vi "lvEtherbone.device_write_single.vi"(0 "eb_socketID":i32, 1 "eb_deviceID":i32, 2 "address":u64 format="%.0x", 4 "data":u64 format="%.0x", 5 "error in (no error)":errorcluster) -> (13 "eb_status":T1, 14 "eb_socketID out":i32, 15 "eb_deviceID out":i32, 19 "error out":errorcluster)   [LabVIEW 2009, in "lvEtherbone.lvlib"]
doc: "This is a wrapper around the routine eb_device_read_write. It performs a single Wishbone write cycle."
uses:
  lvEtherbone.lvlib
  lvEtherbone.lveb_status_t.ctl
  lvEtherbone.eb_mode_t.ctl
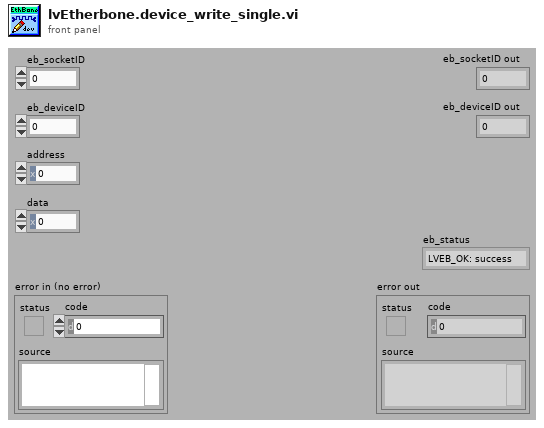
[diagram p1: front panel]
types:
  T1 = typedef "lvEtherbone.lvlib/lvEtherbone.lveb_status_t.ctl" = enum32{"LVEB_OK: success", "LVEB_UNKNOWN: unknown error", "LVEB_OS: operating system forbids access", "LVEB_PORT: port in use or unavailable", "LVEB_ID: ID invalid or out of resources", "LVEB_SOCKET: socket invalid or unavailable", "LVEB_EB: remote address is not Etherbone conformant", "LVEB_IP: bad format or network address", "LVEB_PORTWIDTH: port width error", "LVEB_DEVICEBUSY: Etherbone device still busy", "LVEB_DEVICEFAIL: operation on Wishbone device failed", "LVEB_DEVICEEXIST: Etherbone device already exists, overlaps, or does not exist", "LVEB_TIMEDOUT: a timeout occurred", "LVEB_OVERFLOW: payload of Etherbone exceeded", "LVEB_ADDRESS: bad address", "LVEB_ADDRESSWIDTH: address width error"}
  T2 = typedef "lvEtherbone.lvlib/lvEtherbone.eb_mode_t.ctl" = i32
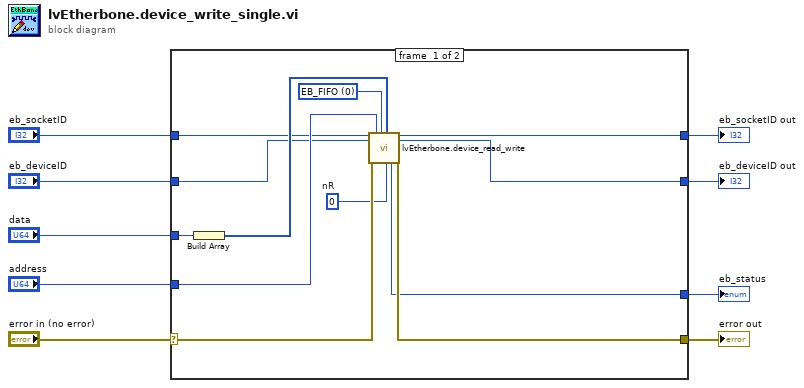
[diagram p0: block diagram]
diagram:
  n1 = case shown="Error" "error in (no error)" {
    selector: "error in (no error)" -> [w17 w24]
    tunnel: [w16 w24] -> w8
    tunnel: "address" -> [w21 _]
    tunnel: "data" -> [w19 _]
    tunnel: "eb_socketID" -> [w15 w23]
    tunnel: [w14 w23] -> w4
    tunnel: "eb_deviceID" -> [w13 w22]
    tunnel: [w12 w22] -> w2
    tunnel: [w10 _] -> w1
    frame #0 {
      w11 = 0  # nR
      w20 = T2 0 items=["EB_UNDEFINED"=-1, "EB_FIFO"=0, "EB_LINEAR"=1] ("modeW")
      n2 = Build Array(w19) -> (w18:u64[])
      n3 = call "lvEtherbone.device_read_write.vi"("eb_socket_ID"=w15, "eb_device_ID"=w13, "error in (no error)"=w17, "addressW"=w21, "modeW"=w20, "dataW"=w18, "nR"=w11) -> ("eb_status"=w10:T1, "eb_socket_ID out"=w14:i32, "eb_device_ID out"=w12:i32, "error out"=w16:errorcluster)  [unwired: 7 in, 2 out]
    }
    frame #1 {
    }
  }
  "error out" <- w8
  "eb_socketID out" <- w4
  "eb_deviceID out" <- w2
  "eb_status" <- w1
